vi "Find frame or struct.vi"(11 "GObj Refnum":refnum<vi>) -> (0 "error IO":errorcluster, 3 "output cluster":T1)   [LabVIEW 2015]
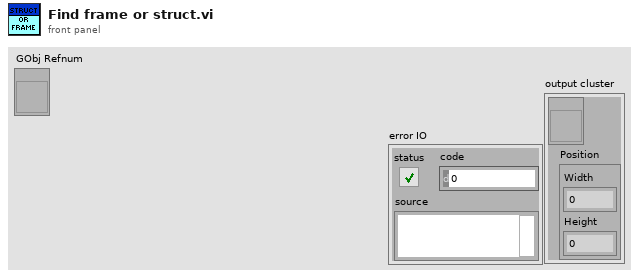
[diagram p1: front panel]
types:
  T1 = cluster{refnum<vi>, "Position":cluster{"Width":dbl, "Height":dbl}}
  T2 = typedef "LVBoundsTypeDef.ctl" = cluster{"Width":u32, "Height":u32}
  T3 = typedef "LVPositionTypeDef.ctl" = cluster{"Left":i32, "Top":i32}
  T4 = cluster{"Gen Refnum":refnum<vi>, "Position":cluster{"Width":dbl, "Height":dbl}}
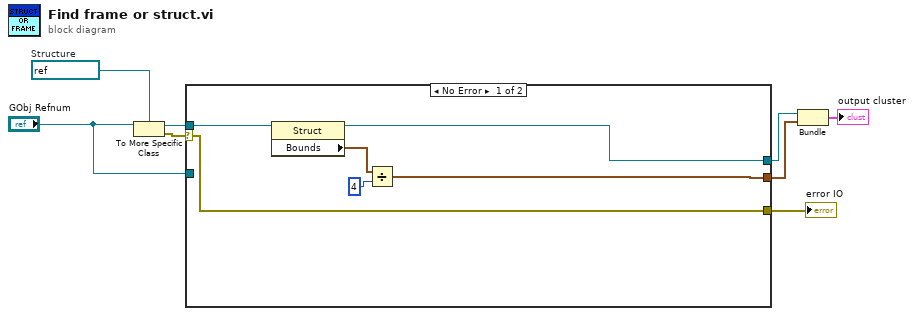
[diagram p0: block diagram]
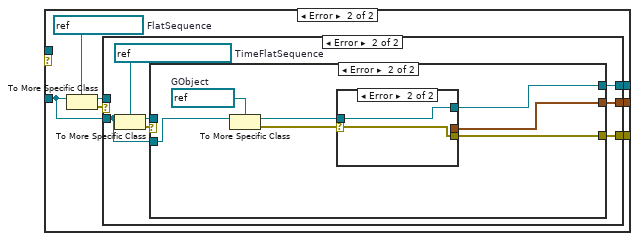
[diagram p2: hidden frame]
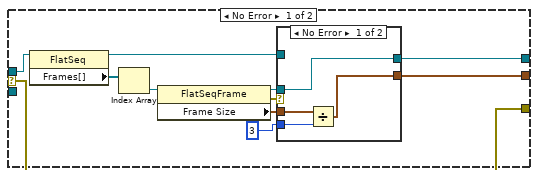
[diagram p3: hidden frame]
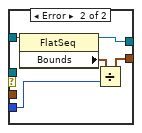
[diagram p4: hidden frame]
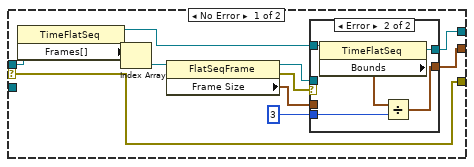
[diagram p5: hidden frame]
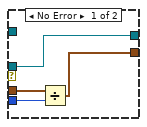
[diagram p6: hidden frame]
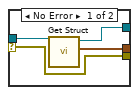
[diagram p7: hidden frame]
diagram:
  w7 = refnum<vi> refnum  # Structure
  n1 = To More Specific Class(target class=w7, reference="GObj Refnum") -> (specific class reference=w8:refnum<vi>, error out=w6:errorcluster)  [unwired: 1 in]
  n2 = case shown="No Error" w6 {
    selector: w6 -> [w11 _]
    tunnel: w8 -> [w14 _]
    tunnel: "GObj Refnum" -> [_ w21]
    tunnel: [w10 w17] -> w4
    tunnel: [w11 w16] -> w5
    tunnel: [w9 w15] -> w3
    frame No Error {
      n3 = property class="Struct"(reference=w14) -> (reference out=w9:refnum<vi>, "Bounds"=w13:T2)  [unwired: 1 in, 1 out]
      n4 = Divide(x=w13, y=4) -> (x/y=w10:cluster{"Width":dbl, "Height":dbl})
    }
    frame Error {
      w18 = refnum<vi> refnum  # FlatSequence
      n5 = To More Specific Class(target class=w18, reference=w21) -> (specific class reference=w19:refnum<vi>, error out=w20:errorcluster)  [unwired: 1 in]
      n6 = case shown="Error" w20 {
        selector: w20 -> [w31 _]
        tunnel: w21 -> [_ w42]
        tunnel: w19 -> [w32 _]
        tunnel: [w27 w45] -> w17
        tunnel: [w31 w44] -> w16
        tunnel: [w23 w43] -> w15
        frame No Error {
          n7 = property class="FlatSeq"(reference=w32) -> (reference out=w22:refnum<vi>, "Frames[]"=w30:refnum<vi>[])  [unwired: 1 in, 1 out]
          n8 = Index Array(array=w30) -> (element=w29:refnum<vi>)  [unwired: 1 in]
          n9 = property class="FlatSeqFrame"(reference=w29) -> (reference out=w24:refnum<vi>, error out=w25:errorcluster, "Frame Size"=w28:T2)  [unwired: 1 in]
          n10 = case shown="No Error" w25 {
            tunnel: 3 -> [w33 w38]
            tunnel: w28 -> [w36 _]
            tunnel: [w35 w37] -> w27
            tunnel: w24 -> [w34 _]
            tunnel: [w34 w40] -> w23
            tunnel: w22 -> [_ w41]
            frame No Error {
              n11 = Divide(x=w36, y=w33) -> (x/y=w35:cluster{"Width":dbl, "Height":dbl})
            }
            frame Error {
              n12 = property class="FlatSeq"(reference=w41) -> (reference out=w40:refnum<vi>, "Bounds"=w39:T2)  [unwired: 1 in, 1 out]
              n13 = Divide(x=w39, y=w38) -> (x/y=w37:cluster{"Width":dbl, "Height":dbl})
            }
          }
        }
        frame Error {
          w48 = refnum<vi> refnum  # TimeFlatSequence
          n14 = To More Specific Class(target class=w48, reference=w42) -> (specific class reference=w46:refnum<vi>, error out=w47:errorcluster)  [unwired: 1 in]
          n15 = case shown="Error" w47 {
            selector: w47 -> [w50 _]
            tunnel: w46 -> [w57 _]
            tunnel: [w53 w69] -> w45
            tunnel: [w50 w71] -> w44
            tunnel: [w49 w73] -> w43
            tunnel: w42 -> [_ w70]
            frame No Error {
              n16 = property class="TimeFlatSeq"(reference=w57) -> (reference out=w54:refnum<vi>, "Frames[]"=w59:refnum<vi>[])  [unwired: 1 in, 1 out]
              n17 = Index Array(array=w59) -> (element=w58:refnum<vi>)  [unwired: 1 in]
              n18 = property class="FlatSeqFrame"(reference=w58) -> (reference out=w55:refnum<vi>, error out=w56:errorcluster, "Frame Size"=w52:T2)  [unwired: 1 in]
              n19 = case shown="Error" w56 {
                tunnel: w52 -> [w61 _]
                tunnel: [w63 w65] -> w53
                tunnel: w55 -> [w62 _]
                tunnel: [w62 w67] -> w49
                tunnel: w54 -> [_ w68]
                tunnel: 3 -> [w60 w64]
                frame No Error {
                  n20 = Divide(x=w61, y=w60) -> (x/y=w63:cluster{"Width":dbl, "Height":dbl})
                }
                frame Error {
                  n21 = property class="TimeFlatSeq"(reference=w68) -> (reference out=w67:refnum<vi>, "Bounds"=w66:T2)  [unwired: 1 in, 1 out]
                  n22 = Divide(x=w66, y=w64) -> (x/y=w65:cluster{"Width":dbl, "Height":dbl})
                }
              }
            }
            frame Error {
              w75 = refnum<vi> refnum  # GObject
              n23 = To More Specific Class(target class=w75, reference=w70) -> (specific class reference=w74:refnum<vi>, error out=w72:errorcluster)  [unwired: 1 in]
              n24 = case shown="Error" w72 {
                selector: w72 -> [w77 w81]
                tunnel: w74 -> [w79 w80]
                tunnel: [w78 w80] -> w73
                tunnel: [w77 w81] -> w71
                tunnel: [w76 _] -> w69
                frame No Error {
                  n25 = call <resource>:"Get Struct.vi"("reference"=w79) -> ("Position"=w76:T3, "Gen Refnum"=w78:refnum<vi>)  [unwired: 9 in]
                }
                frame Error {
                }
              }
            }
          }
        }
      }
    }
  }
  "error IO" <- w5
  n26 = Bundle("Gen Refnum"=w3, "Position"=w4) -> (→"output cluster":T4)  [unwired: 1 in]
